vi "read device xml data.vi"(8 "error in (no error)":errorcluster, 11 "TCP Network Connection in":refnum<k5>) -> (0 "error out":errorcluster, 2 "data out":string, 3 "TCP Network Connection out":refnum<k5>)   [LabVIEW 2020]
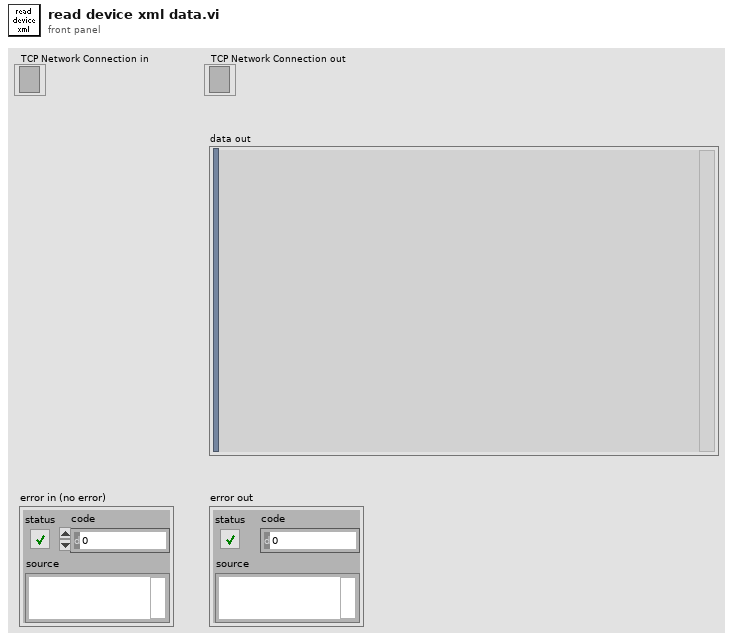
[diagram p1: front panel]
types:
  T1 = enum16{"big-endian, network order", "native, host order", "little-endian"}
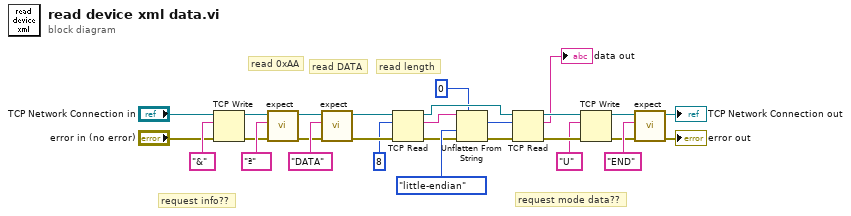
[diagram p0: block diagram]
diagram:
  # "request mode data??"
  # "request info??"
  # "read length"
  # "read DATA"
  # "read 0xAA"
  n1 = TCP Write(connection ID="TCP Network Connection in", data in="&", error in (no error)="error in (no error)") -> (connection ID out=w5:refnum<k5>, error out=w4:errorcluster)  [unwired: 1 in, 1 out]
  n2 = call "expect.vi"("error in (no error)"=w4, "data expected"="ª" ("data in"), "TCP Network Connection in"=w5) -> ("error out"=w7:errorcluster, "TCP Network Connection out"=w10:refnum<k5>)  [unwired: 6 in, 1 out]
  n3 = call "expect.vi"("error in (no error)"=w7, "data expected"="DATA" ("data in"), "TCP Network Connection in"=w10) -> ("error out"=w9:errorcluster, "TCP Network Connection out"=w11:refnum<k5>)  [unwired: 6 in, 1 out]
  n4 = TCP Read(connection ID=w11, bytes to read=8, error in (no error)=w9) -> (connection ID out=w18:refnum<k5>, data out=w15:string, error out=w13:errorcluster)  [unwired: 2 in]
  n5 = Unflatten From String(type=0 ("bytes to read"), binary string=w15, byte order (0:big-endian, network order)=T1."little-endian", error in (no error)=w13) -> (value=w19:i32, error out=w14:errorcluster)  [unwired: 1 in, 1 out]
  n6 = TCP Read(connection ID=w18, bytes to read=w19, error in (no error)=w14) -> (connection ID out=w22:refnum<k5>, data out=→"data out":string, error out=w23:errorcluster)  [unwired: 2 in]
  n7 = TCP Write(connection ID=w22, data in="U", error in (no error)=w23) -> (connection ID out=w25:refnum<k5>, error out=w24:errorcluster)  [unwired: 1 in, 1 out]
  n8 = call "expect.vi"("error in (no error)"=w24, "data expected"="END" ("data in"), "TCP Network Connection in"=w25) -> ("error out"=→"error out":errorcluster, "TCP Network Connection out"=→"TCP Network Connection out":refnum<k5>)  [unwired: 6 in, 1 out]
